vi "GEN_TimerPerS.vi"(9 "Data_In":T1={"Value"=0.0, "GUI Data Cluster"={"SBR"=0}, "Timing"={"Last Operation"=0.0, "Stop @ T"=FALSE, "Delta T Log"=FALSE, "End T"=0.0, "Delta T"=0.0, "Last Temp"=0.0}, "Measurements"=[], "Hardware"={"VNA TCP Con"=refnum, "VNA TCP Port"=5025, "Global T VAR"="", "Global B VAR"=""}, "Operation"={"Operation Mode"=enum."Logging", "Status"="", "NewLog?"=FALSE}} {"GUI Data Cluster"."SBR" format="%08b"}, 10 "Config_In":T4={"General"={"Config.ini"=path "", "Default Logging Path"=path ""}, "Hardware"={"Measure Rate (1/s)"=0, "HP DMM VISA"="", "LS 335 VISA"="", "HP DM"={"Range"=enum."Autorange", "Autozero"=FALSE, "Display"=enum."3 1/2 Digit", "Blank LCD"=FALSE}}, "Operation"={"Operation Mode"=enum."Idle-Off", "Status"="", "NewLog?"=FALSE, "OvenWarn"=FALSE}}) -> (0 "Time":bool, 1 "Data_In 2":T1={"Value"=0.0, "GUI Data Cluster"={"SBR"=0}, "Timing"={"Last Operation"=0.0, "Stop @ T"=FALSE, "Delta T Log"=FALSE, "End T"=0.0, "Delta T"=0.0, "Last Temp"=0.0}, "Measurements"=[], "Hardware"={"VNA TCP Con"=refnum, "VNA TCP Port"=5025, "Global T VAR"="", "Global B VAR"=""}, "Operation"={"Operation Mode"=enum."Logging", "Status"="", "NewLog?"=FALSE}} {"GUI Data Cluster"."SBR" format="%08b"}, 2 "Config_In 2":T4={"General"={"Config.ini"=path "", "Default Logging Path"=path ""}, "Hardware"={"Measure Rate (1/s)"=0, "HP DMM VISA"="", "LS 335 VISA"="", "HP DM"={"Range"=enum."Autorange", "Autozero"=FALSE, "Display"=enum."3 1/2 Digit", "Blank LCD"=FALSE}}, "Operation"={"Operation Mode"=enum."Idle-Off", "Status"="", "NewLog?"=FALSE, "OvenWarn"=FALSE}})   [LabVIEW 2021]
uses:
  Data_Cluster.ctl
  Mode_Enum.ctl
  Config_Cluster.ctl
  Measurement_Cluster.ctl
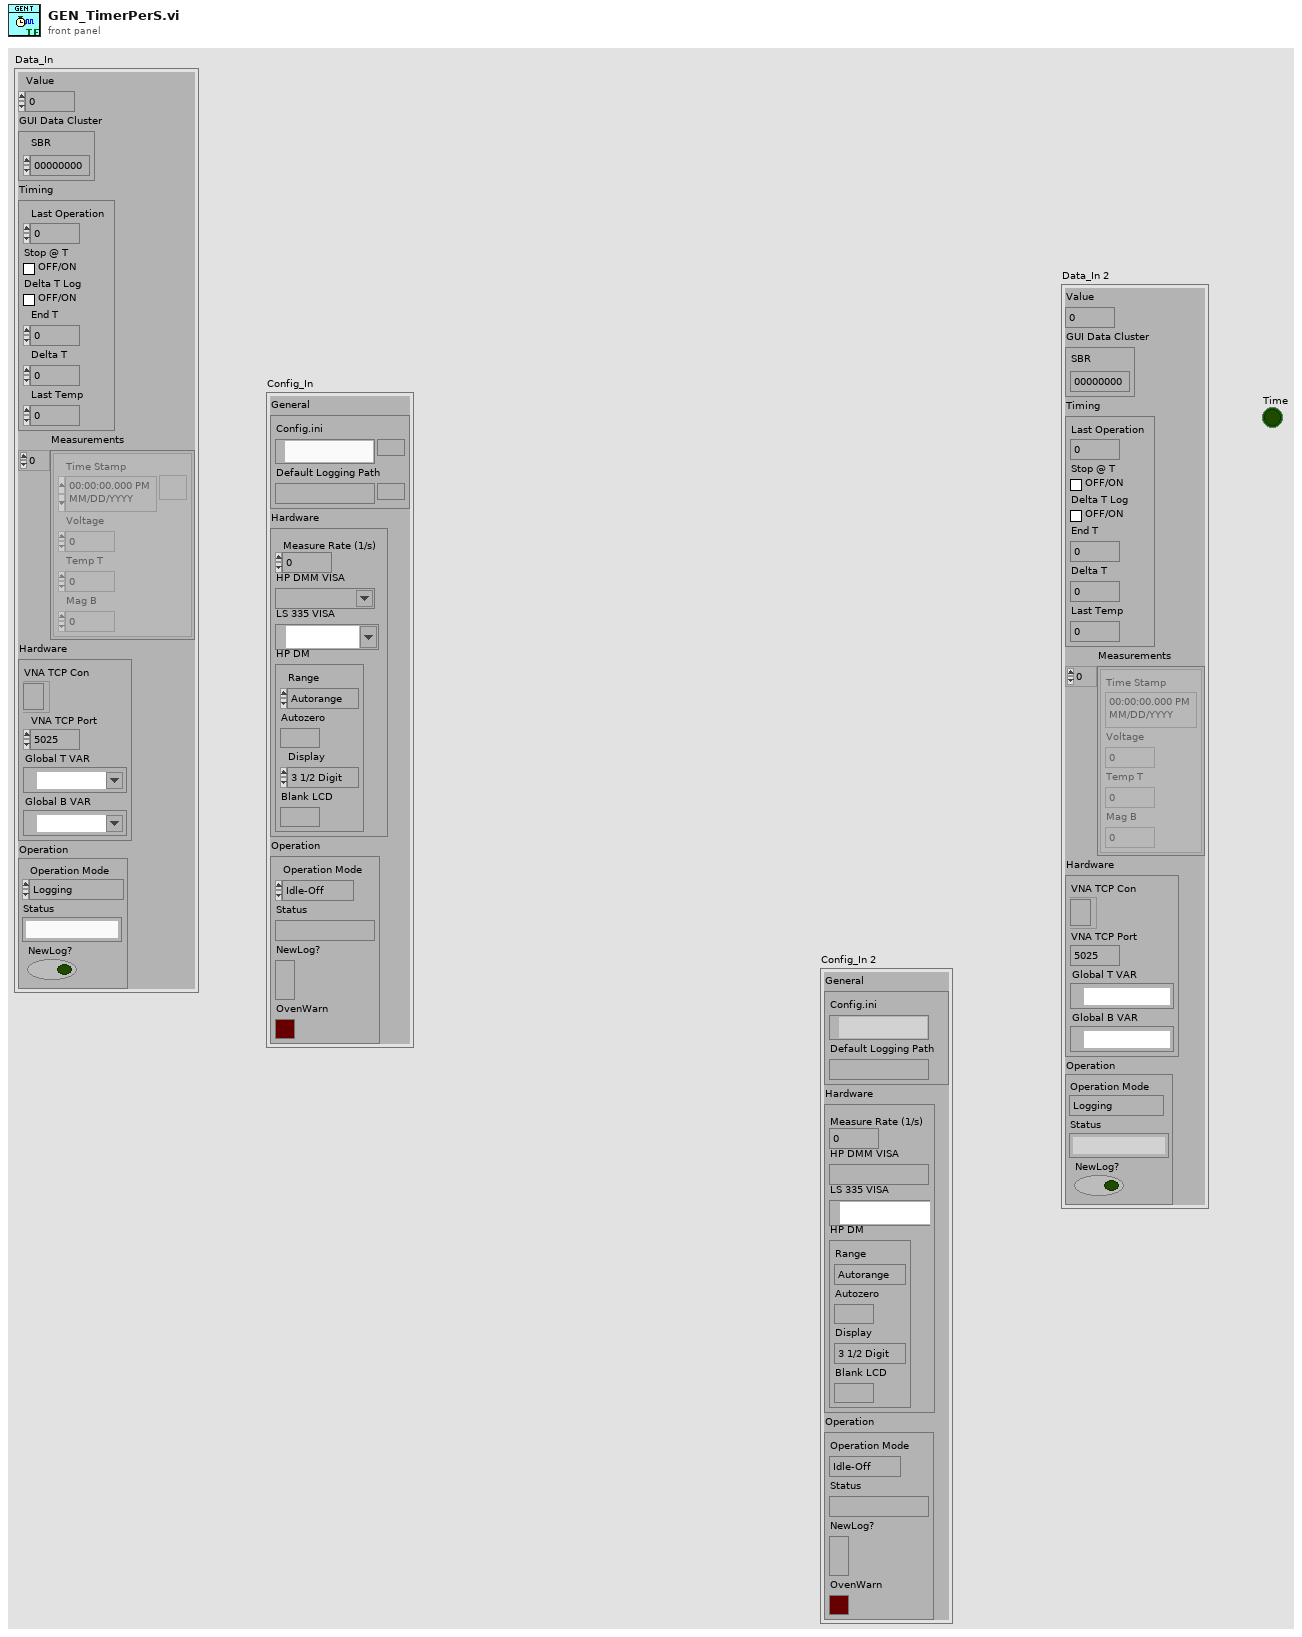
[diagram p1: front panel]
types:
  T1 = typedef "Data_Cluster.ctl" = cluster{"Value":dbl, "GUI Data Cluster":cluster{"SBR":u16}, "Timing":cluster{"Last Operation":dbl, "Stop @ T":bool, "Delta T Log":bool, "End T":dbl, "Delta T":dbl, "Last Temp":dbl}, "Measurements":T2[], "Hardware":cluster{"VNA TCP Con":refnum<k5>, "VNA TCP Port":i32, "Global T VAR":refnum<k21>, "Global B VAR":refnum<k21>}, "Operation":cluster{"Operation Mode":T3, "Status":string, "NewLog?":bool}}
  T2 = typedef "Measurement_Cluster.ctl" = cluster{"Time Stamp":timestamp, "Voltage":dbl, "Temp T":dbl, "Mag B":dbl}
  T3 = typedef "Mode_Enum.ctl" = enum16{"OvenNRDY", "Logging", "Idle-Off", "Idle"}
  T4 = typedef "Config_Cluster.ctl" = cluster{"General":cluster{"Config.ini":path, "Default Logging Path":path}, "Hardware":cluster{"Measure Rate (1/s)":i32, "HP DMM VISA":refnum<visa-resource-name>, "LS 335 VISA":refnum<visa-resource-name>, "HP DM":cluster{"Range":enum16{"Autorange", "30mV", "300mV", "3V", "30V"}, "Autozero":bool, "Display":enum16{"3 1/2 Digit", "4 1/2 Digit", "5 1/2 Digit"}, "Blank LCD":bool}}, "Operation":cluster{"Operation Mode":T3, "Status":string, "NewLog?":bool, "OvenWarn":bool}}
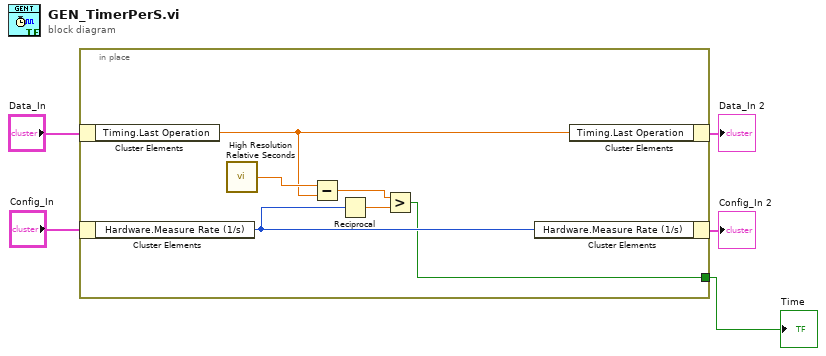
[diagram p0: block diagram]
diagram:
  n1 = in-place {
    in-place-border: [w6] -> w1
    n2 = in-place-cluster #1("Data_In") -> ("Timing.Last Operation"=w9:dbl)
    n3 = in-place-cluster #2("Config_In") -> ("Hardware.Measure Rate (1/s)"=w10:i32)
    n4 = call <vilib>:"High Resolution Relative Seconds.vi"() -> ("relative seconds"=w11:dbl)
    n5 = Subtract(x=w11, y=w9) -> (x-y=w7:dbl)
    n6 = Reciprocal(x=w10) -> (1/x=w8:dbl)
    n7 = Greater?(x=w7, y=w8) -> (0:w6:bool)
    n8 = in-place-cluster #2("Hardware.Measure Rate (1/s)"=w10) -> (→"Config_In 2":T4)
    n9 = in-place-cluster #1("Timing.Last Operation"=w9) -> (→"Data_In 2":T1)
  }
  "Time" <- w1
